vi "test_FPGAWrapper_RAPS.vi"() -> ()   [LabVIEW 2010, in "FPGAWrapperMH120124RAPS_PXI7813R.lvclass"]
uses:
  FPGAWrapperMH120124RAPS_PXI7813R.lvclass
  fpgaVIsAndControls/ellipsoid_parameters_cluster.ctl
  Trajectory/TrajectoryMH100122AODRAPS/TrajectoryMH100122AODRAPS/raps_points_cluster.ctl
  common/classes/ErrorController/ErrorController/ErrorController.lvclass
  common/classes/ErrorController/ErrorController/class_data.vi
  Trajectory/TrajectoryMH100122AODRAPS/TrajectoryMH100122AODRAPS/TrajectoryMH100122AODRAPS.lvclass
panel:
  in  "RAPS points cluster in":T1
  in  "amplitude in":dbl=3400.0
  in  "ellipsoid parameter cluster":T2={"a"=0.0, "b"=0.125, "c"=0.5, "d"=0.015625, "e"=0.5, "k"=0, "width"=0.0} {"a" format="%.16g"; "b" format="%.16g"; "c" format="%.16g"; "d" format="%.16g"}
  in  "AOD bandwidth freq. (Hz)":dbl[unit]=34000000.0
  in  "AOD center freq. (Hz)":dbl[unit]=94000000.0
  in  "AOD equilibration time":dbl[unit]=7e-06
  in  "number of pixels":i64=2
  in  "pixel dwell time":dbl[unit]=4.9999999999999996e-06
  in  "subpattern?":bool
  in  "number of channels":i32=3
  in  "block size":i32=10000
  out "channel data block":dbl[][](graph)
  in  "timeout (ms)":i32=500
  out "timed out?":bool
  out "samples read":i32
  in  "button:run":bool
  out "FPGAWrapper":refnum<class "FPGAWrapperMH120124RAPS_PXI7813R.lvclass">
  in  "button:create":bool
  in  "button:stop":bool
  out "error controller loaded?":bool=TRUE
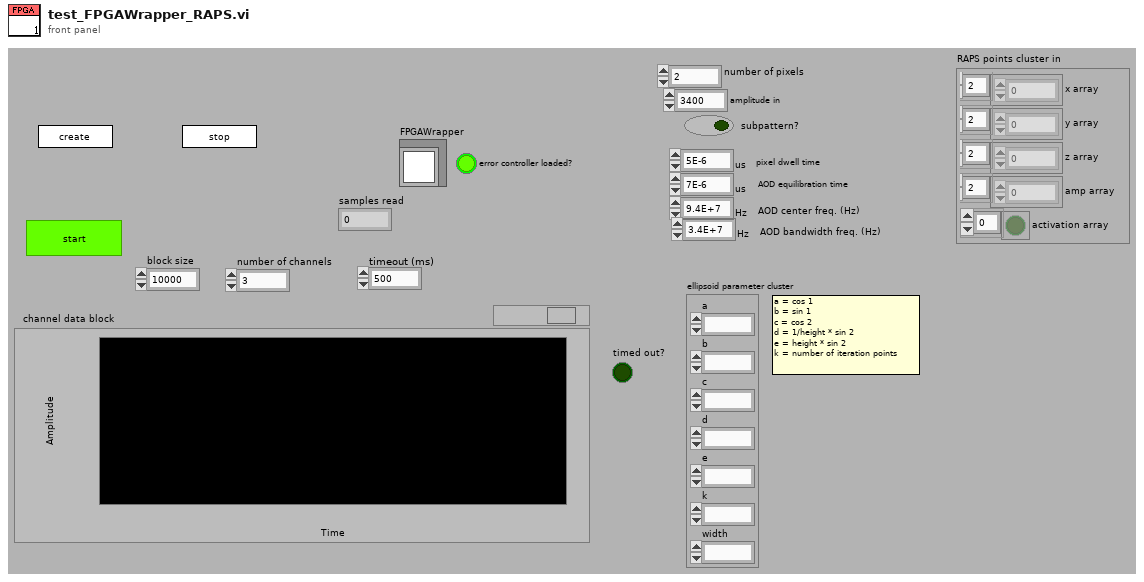
[diagram p1: front panel]
types:
  T1 = typedef "TrajectoryMH100122AODRAPS.lvclass/raps_points_cluster.ctl" = cluster{"x array":u16[], "y array":u16[], "z array":u16[], "amp array":u16[], "activation array":bool[]}
  T2 = typedef "ellipsoid_parameters_cluster.ctl" = cluster{"a":fxp<+/-,16,1>, "b":fxp<+/-,16,1>, "c":fxp<+/-,16,1>, "d":fxp<+/-,16,1>, "e":fxp<+/-,24,16>, "k":u16, "width":fxp<+,16,16>}
  T3 = typedef "plugin_specification.ctl" = cluster{"class path":string, "configuration":string, "label":string, "settings name":string}
  T4 = typedef "XComponentSpecification.xctl/data.ctl" = cluster{"class path":string, "configuration":string, "label":string, "settings name":string}
  T5 = typedef "pixel_raw_data_array.ctl" = dbl[][]
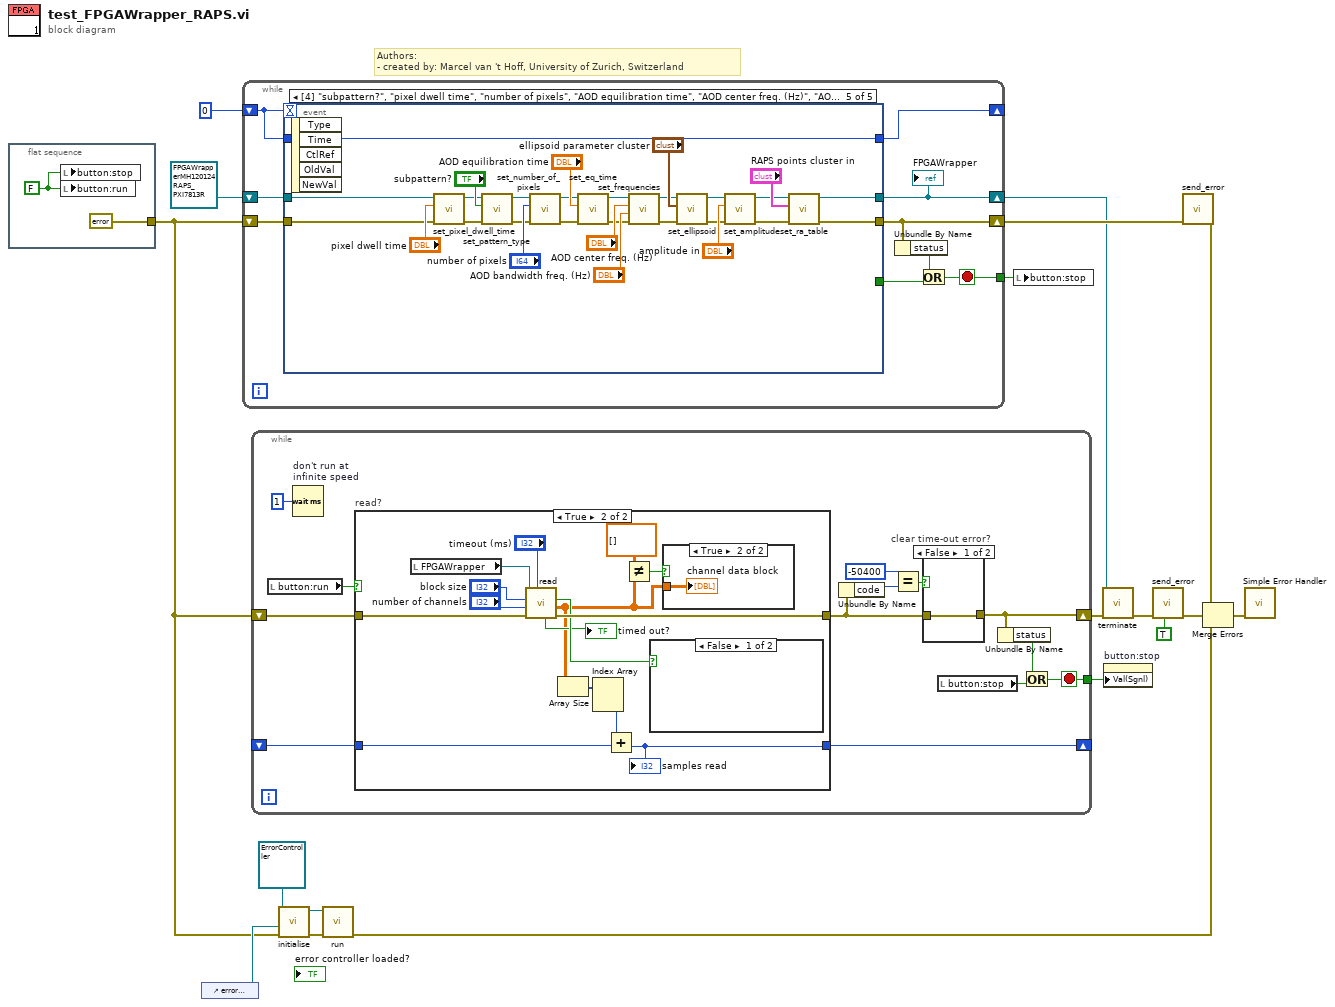
[diagram p0: block diagram]
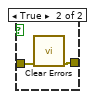
[diagram p2: hidden frame]
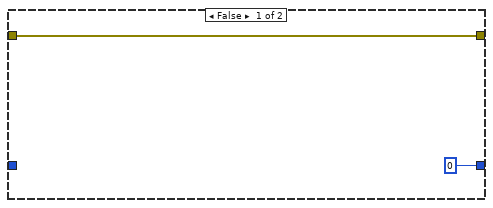
[diagram p3: hidden frame]
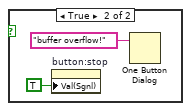
[diagram p4: hidden frame]
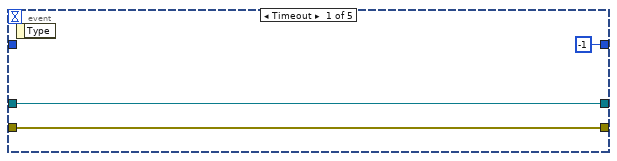
[diagram p6: hidden frame]
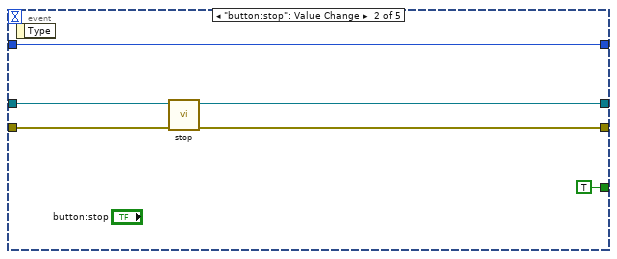
[diagram p7: hidden frame]
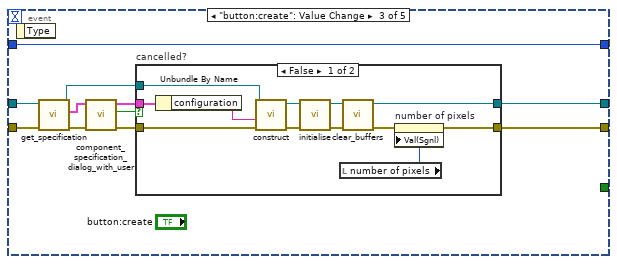
[diagram p8: hidden frame]
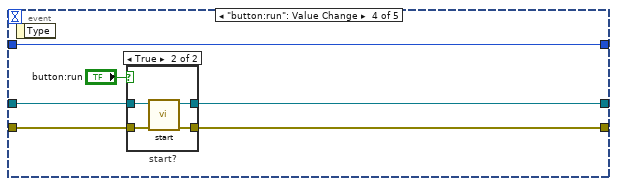
[diagram p10: hidden frame]
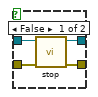
[diagram p11: hidden frame]
diagram:
  # "Authors: \n- created by: Marcel van 't Hoff, University of Zurich, Switzerland"
  n1 = flat-sequence {
    tunnel: [errorcluster {"status"=FALSE, "code"=0, "source"=""} ("error in (no error)")] -> w11
    frame #0 {
      w19 = FALSE ("button:stop")
      n2 = local write "button:stop"(w19) -> ()
      n3 = local write "button:run"(w19) -> ()
    }
  }
  n4 = control-ref of="error controller loaded?"() -> (w18:refnum<vi>)
  n5 = while {
    shift-right: [w28] -> w8
    shift-left: refnum<class "FPGAWrapperMH120124RAPS_PXI7813R.lvclass"> refnum ("FPGAWrapperMH120124RAPS_PXI7813R.lvclass") -> [w29]
    shift-right: [w26] -> _
    shift-left: 0 -> [w27]
    shift-right: [w24] -> w12
    shift-left: w11 -> [w25]
    tunnel: [w21] -> w1
    stop <- w21 stop-if-true
    n6 = event shown="[4] \"subpattern?\", \"pixel dwell time\", \"number of pixels\", \"AOD equilibration time\", \"AOD center freq. (Hz)\", \"AOD bandwidth freq. (Hz)\", \"ellipsoid parameter cluster\", \"amplitude in\": Value Change" {
      selector: _ -> [_ _ _ _ _]
      dyn-events: _ -> [_ _ _ _ _]
      timeout: w27 -> [_ _ _ _ _]
      tunnel: w29 -> [w32 w34 w40 w66 w86]
      tunnel: [w32 w33 w39 w65 w80] -> w28
      tunnel: w27 -> [_ w38 w49 w69 w105]
      tunnel: [-1 w38 w49 w69 w105] -> w26
      tunnel: [w30 w35 w41 w64 w78] -> w24
      tunnel: w25 -> [w30 w36 w47 w68 w85]
      tunnel: [_ TRUE _ _ _] -> w22
      event Timeout {
        n7 = event-data() -> ()  [unwired: 1 in, 1 out]
      }
      event "button:stop": Value Change {
        n8 = event-data() -> ()  [unwired: 1 in, 1 out]
        n9 = call-dynamic "stop.vi"("error in (no error)"=w36, "FPGAWrapperMH120124RAPS_PXI7813R in"=w34) -> ("error out"=w35:errorcluster, "FPGAWrapperMH120124RAPS_PXI7813R out"=w33:refnum<class "FPGAWrapperMH120124RAPS_PXI7813R.lvclass">)  [unwired: 8 out]
      }
      event "button:create": Value Change {
        n10 = event-data() -> ()  [unwired: 1 in, 1 out]
        n11 = call-dynamic "get_specification.vi"("error in (no error)"=w47, "GenericPlugin in"=w40) -> ("error out"=w48:errorcluster, "component specification"=w46:T3, "GenericPlugin out"=w42:refnum<class "FPGAWrapperMH120124RAPS_PXI7813R.lvclass">)  [unwired: 6 in, 1 out]
        n12 = call "component_specification_dialog_with_user.vi"("error in (no error)"=w48, "component specification in"=w46) -> ("error out"=w44:errorcluster, "cancelled?"=w45:bool, "component specification out"=w43:T4)  [unwired: 7 in]
        n13 = case "cancelled?" shown="False" w45 {
          tunnel: w44 -> [w60 w63]
          tunnel: w43 -> [w61 _]
          tunnel: w42 -> [w57 w62]
          tunnel: [w50 w63] -> w41
          tunnel: [w53 w62] -> w39
          frame False {
            n14 = Unbundle By Name(w61) -> ("configuration"=w54:string)
            n15 = call-dynamic "construct.vi"("error in (no error)"=w60, "configuration name"=w54, "GenericPlugin in"=w57) -> ("error out"=w59:errorcluster, "GenericPlugin out"=w56:refnum<class "FPGAWrapperMH120124RAPS_PXI7813R.lvclass">)  [unwired: 7 in]
            n16 = call-dynamic "initialise.vi"("error in (no error)"=w59, "GenericPlugin in"=w56) -> ("error out"=w58:errorcluster, "GenericPlugin out"=w55:refnum<class "FPGAWrapperMH120124RAPS_PXI7813R.lvclass">)  [unwired: 1 in, 7 out]
            n17 = local read "number of pixels"() -> (w52:i64)
            n18 = call-dynamic "clear_buffers.vi"("error in (no error)"=w58, "FPGAWrapperMH120124RAPS_PXI7813R in"=w55) -> ("error out"=w51:errorcluster, "FPGAWrapperMH120124RAPS_PXI7813R out"=w53:refnum<class "FPGAWrapperMH120124RAPS_PXI7813R.lvclass">)  [unwired: 8 in]
            n19 = property on="number of pixels" class="DigNum (strict)"(error in=w51, "Val(Sgnl)"=w52) -> (error out=w50:errorcluster)  [unwired: 1 in, 1 out]
          }
          frame True {
          }
        }
      }
      event "button:run": Value Change {
        n20 = event-data() -> ()  [unwired: 1 in, 1 out]
        n21 = case "start?" shown="True" "button:run" {
          tunnel: w68 -> [w73 w77]
          tunnel: w66 -> [w72 w76]
          tunnel: [w71 w75] -> w65
          tunnel: [w70 w74] -> w64
          frame False {
            n22 = call-dynamic "stop.vi"("error in (no error)"=w73, "FPGAWrapperMH120124RAPS_PXI7813R in"=w72) -> ("error out"=w70:errorcluster, "FPGAWrapperMH120124RAPS_PXI7813R out"=w71:refnum<class "FPGAWrapperMH120124RAPS_PXI7813R.lvclass">)  [unwired: 8 out]
          }
          frame True {
            n23 = call-dynamic "start.vi"("error in (no error)"=w77, "FPGAWrapperMH120124RAPS_PXI7813R in"=w76) -> ("error out"=w74:errorcluster, "FPGAWrapperMH120124RAPS_PXI7813R out"=w75:refnum<class "FPGAWrapperMH120124RAPS_PXI7813R.lvclass">)  [unwired: 8 out]
          }
        }
      }
      event "subpattern?", "pixel dwell time", "number of pixels", "AOD equilibration time", "AOD center freq. (Hz)", "AOD bandwidth freq. (Hz)", "amplitude in": Value Change {
        n24 = event-data() -> ()  [unwired: 1 in, 5 out]
        n25 = call-dynamic "set_pixel_dwell_time.vi"("error in (no error)"=w85, "pixel dwell time"="pixel dwell time", "FPGAWrapperMH120124RAPS_PXI7813R in"=w86) -> ("error out"=w96:errorcluster, "FPGAWrapperMH120124RAPS_PXI7813R out"=w87:refnum<class "FPGAWrapperMH120124RAPS_PXI7813R.lvclass">)  [unwired: 7 in]
        n26 = call-dynamic "set_pattern_type.vi"("error in (no error)"=w96, "subpattern?"="subpattern?", "FPGAWrapperMH120124RAPS_PXI7813R in"=w87) -> ("error out"=w95:errorcluster, "FPGAWrapperMH120124RAPS_PXI7813R out"=w88:refnum<class "FPGAWrapperMH120124RAPS_PXI7813R.lvclass">)  [unwired: 7 in]
        n27 = call-dynamic "set_number_of_pixels.vi"("error in (no error)"=w95, "number of pixels"="number of pixels", "FPGAWrapperMH120124RAPS_PXI7813R in"=w88) -> ("error out"=w84:errorcluster, "FPGAWrapperMH120124RAPS_PXI7813R out"=w83:refnum<class "FPGAWrapperMH120124RAPS_PXI7813R.lvclass">)  [unwired: 7 in]
        n28 = call-dynamic "set_eq_time.vi"("error in (no error)"=w84, "AOD equilibration time"="AOD equilibration time", "FPGAWrapperMH120124RAPS_PXI7813R in"=w83) -> ("error out"=w94:errorcluster, "FPGAWrapperMH120124RAPS_PXI7813R out"=w89:refnum<class "FPGAWrapperMH120124RAPS_PXI7813R.lvclass">)  [unwired: 7 in]
        n29 = call-dynamic "set_frequencies.vi"("error in (no error)"=w94, "AOD bandwidth freq. (Hz)"="AOD bandwidth freq. (Hz)", "AOD center freq. (Hz)"="AOD center freq. (Hz)", "FPGAWrapperMH120124RAPS_PXI7813R in"=w89) -> ("error out"=w93:errorcluster, "FPGAWrapperMH120124RAPS_PXI7813R out"=w90:refnum<class "FPGAWrapperMH120124RAPS_PXI7813R.lvclass">)  [unwired: 6 in]
        n30 = call-dynamic "set_ellipsoid.vi"("error in (no error)"=w93, "ellipsoid parameter cluster"="ellipsoid parameter cluster", "FPGAWrapperMH120124RAPS_PXI7813R in"=w90) -> ("error out"=w92:errorcluster, "FPGAWrapperMH120124RAPS_PXI7813R out"=w91:refnum<class "FPGAWrapperMH120124RAPS_PXI7813R.lvclass">)  [unwired: 7 in]
        n31 = call-dynamic "set_amplitude.vi"("error in (no error)"=w92, "amplitude in"="amplitude in", "FPGAWrapperMH120124RAPS_PXI7813R in"=w91) -> ("error out"=w79:errorcluster, "FPGAWrapperMH120124RAPS_PXI7813R out"=w81:refnum<class "FPGAWrapperMH120124RAPS_PXI7813R.lvclass">)  [unwired: 7 in]
        n32 = call-dynamic "set_ra_table.vi"("error in (no error)"=w79, "RAPS points cluster in"="RAPS points cluster in", "FPGAWrapperMH120124RAPS_PXI7813R in"=w81) -> ("error out"=w78:errorcluster, "FPGAWrapperMH120124RAPS_PXI7813R out"=w80:refnum<class "FPGAWrapperMH120124RAPS_PXI7813R.lvclass">)  [unwired: 7 in]
      }
    }
    "FPGAWrapper" <- w28
    n33 = Unbundle By Name(w24) -> ("status"=w23:bool)
    n34 = Or(x=w23, y=w22) -> (x .or. y?=w21:bool)
  }
  n35 = while {
    shift-right: [w117] -> _
    shift-left: _ -> [w116]
    shift-right: [w110] -> w9
    shift-left: w11 -> [w118]
    tunnel: [w109] -> w10
    stop <- w109 stop-if-true
    n36 = local read "button:run"() -> (w107:bool)
    n37 = Wait (ms) "don't run at \ninfinite speed"(milliseconds to wait=u32 1) -> ()  [unwired: 1 out]
    n38 = case "read?" shown="True" w107 {
      tunnel: w118 -> [w123 w138]
      tunnel: [w123 w137] -> w108
      tunnel: w116 -> [_ w129]
      tunnel: [0 w126] -> w117
      frame False {
      }
      frame True {
        n39 = local read "FPGAWrapper"() -> (w124:refnum<class "FPGAWrapperMH120124RAPS_PXI7813R.lvclass">)
        n40 = call-dynamic "read.vi"("timeout (ms)"="timeout (ms)", "error in (no error)"=w138, "number of channels"="number of channels", "block size"="block size", "FPGAWrapperMH120124RAPS_PXI7813R in"=w124) -> ("error out"=w137:errorcluster, "channels raw data block"=w128:T5, "FIFO full?"=w132:bool, "timed out?"=→"timed out?":bool)  [unwired: 3 out]
        n41 = Array Size(array=w128) -> (size(s)=w127:i32[])
        n42 = Index Array(array=w127) -> (element #2=w125:i32)  [unwired: 2 in, 1 out]
        n43 = Add(x=w125, y=w129) -> (x+y=w126:i32)
        "samples read" <- w126
        n44 = Not Equal?(x=dbl[][] [], y=w128) -> (x != y?=w134:bool)
        n45 = case shown="False" w132 {
          frame False {
          }
          frame True {
            n46 = property on="button:stop" class="Bool (strict)"("Val(Sgnl)"=TRUE) -> ()  [unwired: 2 in, 2 out]
            n47 = One Button Dialog(message="buffer overflow!") -> ()  [unwired: 1 in, 1 out]
          }
        }
        n48 = case shown="True" w134 {
          tunnel: w128 -> [_ w141]
          frame False {
          }
          frame True {
            "channel data block" <- w141
          }
        }
      }
    }
    n49 = Unbundle By Name(w108) -> ("code"=w112:i32)
    n50 = Equal?(x=-50400, y=w112) -> (x = y?=w114:bool)
    n51 = case "clear time-out error?" shown="False" w114 {
      tunnel: w108 -> [w119 w121]
      tunnel: [w119 w120] -> w110
      frame False {
      }
      frame True {
        n52 = call <vilib>:"Clear Errors.vi"("error in (no error)"=w121) -> ("error out"=w120:errorcluster)  [unwired: 6 out]
      }
    }
    n53 = local read "button:stop"() -> (w111:bool)
    n54 = Unbundle By Name(w110) -> ("status"=w115:bool)
    n55 = Or(x=w115, y=w111) -> (x .or. y?=w109:bool)
  }
  n56 = call-dynamic "initialise.vi"("error in (no error)"=w11, "error boolean"=w18, "ErrorController in"=refnum<class "ErrorController.lvclass"> refnum) -> ("error out"=w15:errorcluster, "ErrorController out"=w16:refnum<class "ErrorController.lvclass">)  [unwired: 7 in]
  n57 = call "run.vi"("error in (no error)"=w15, "ErrorController in"=w16) -> ("error out"=w3:errorcluster)  [unwired: 8 in, 1 out]
  n58 = local write "button:stop"(w1) -> ()
  n59 = call-dynamic "terminate.vi"("error in (no error)"=w9, "GenericPlugin in"=w8) -> ("error out"=w7:errorcluster)  [unwired: 8 in, 1 out]
  n60 = property on="button:stop" class="Bool (strict)"("Val(Sgnl)"=w10) -> ()  [unwired: 2 in, 2 out]
  n61 = call "send_error.vi"("last error? (F)"=TRUE, "error in (no error)"=w7) -> ("error out"=w5:errorcluster)  [unwired: 9 in]
  n62 = call "send_error.vi"("error in (no error)"=w12) -> ("error out"=w4:errorcluster)  [unwired: 10 in]
  n63 = Merge Errors(w4, w5, w3) -> (w2:errorcluster)
  n64 = call <vilib>:"Simple Error Handler.vi"("error in (no error)"=w2) -> ()  [unwired: 1 in, 8 out]
